vi "DataStorageCloseEventRequest_Create.vi"(7 "Header":T3, 8 "error in (no error)":errorcluster, 9 "DataStorageCloseEventRequest":T1, 10 "IRoutingSource":T2, 11 "ReplyTo":string) -> (0 "error out":errorcluster, 3 "Message":T5)   [LabVIEW 2017]
uses:
  <vilib>/addons/InsightCM/MessageBus/Base/controls/Message.ctl
  <vilib>/addons/InsightCM/MessageBus/Base/controls/MessageHeader.ctl
  <vilib>/addons/InsightCM/MessageBus/Base/controls/KeyValuePair.ctl
  <vilib>/addons/InsightCM/MessageBus/Base/controls/IRoutingSource.ctl
  <vilib>/addons/InsightCM/MessageBus/MessageLibrary/DataStorage/controls/DataStorageCloseEventRequestBody.ctl
  <vilib>/addons/InsightCM/MessageBus/Base/controls/MessageClassType.ctl
  <vilib>/addons/InsightCM/Utilities/PropertyHelpers/PropertyHelpers.lvlib
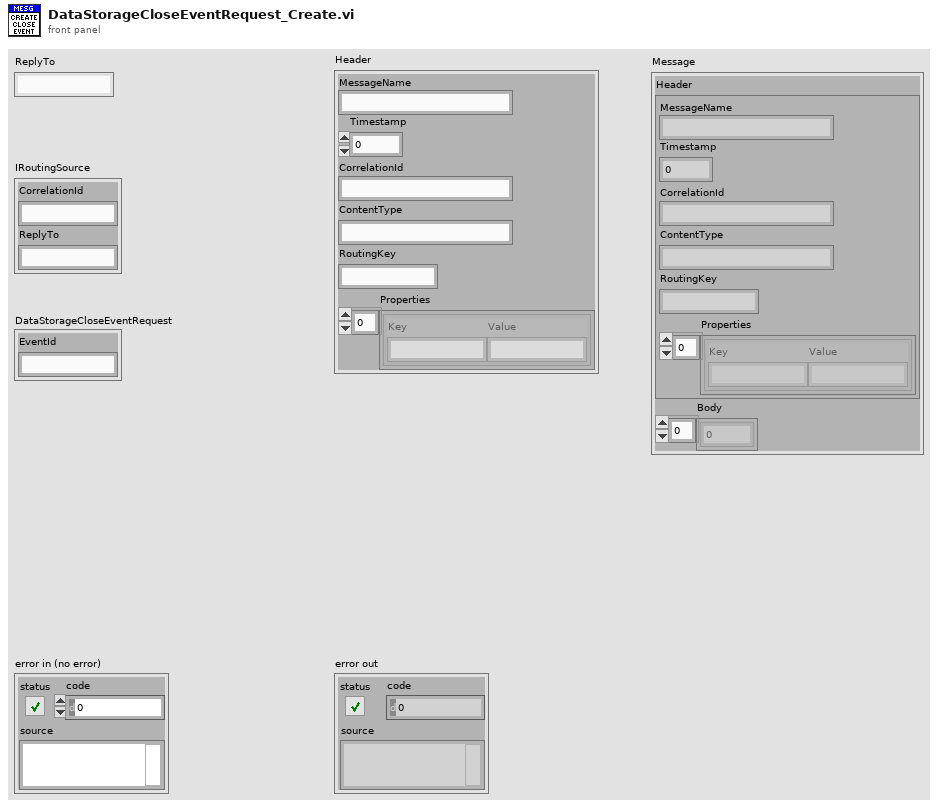
[diagram p1: front panel]
types:
  T1 = typedef "DataStorageCloseEventRequestBody.ctl" = cluster{"EventId":string}
  T2 = typedef "IRoutingSource.ctl" = cluster{"CorrelationId":string, "ReplyTo":string}
  T3 = typedef "MessageHeader.ctl" = cluster{"MessageName":string, "Timestamp":i64, "CorrelationId":string, "ContentType":string, "RoutingKey":string, "Properties":T4[]}
  T4 = typedef "KeyValuePair.ctl" = cluster{"Key":string, "Value":string}
  T5 = typedef "Message.ctl" = cluster{"Header":T3, "Body":u8[]}
  T6 = typedef "MessageClassType.ctl" = enum16{"Request", "Response", "Broadcast", "RoutedMessage"}
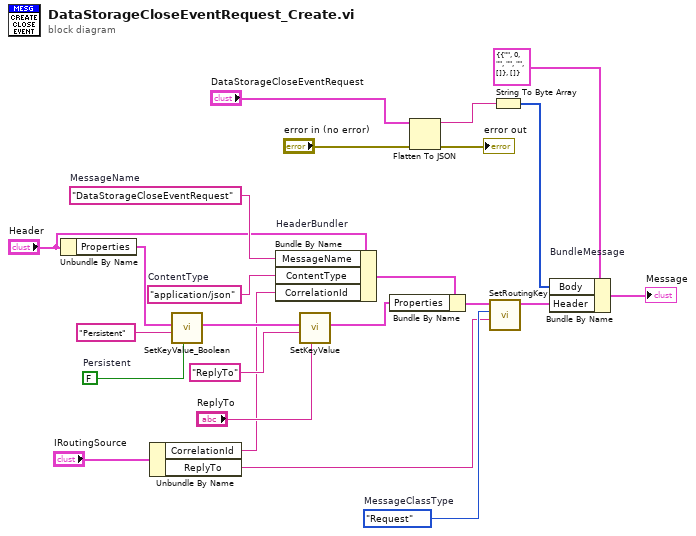
[diagram p0: block diagram]
diagram:
  w20 = MessageClassType."Request"  # MessageClassType
  w15 = FALSE  # Persistent
  w21 = "DataStorageCloseEventRequest"  # MessageName
  w18 = "application/json"  # ContentType
  n1 = Unbundle By Name("Header") -> ("Properties"=w17:T4[])
  n2 = Unbundle By Name("IRoutingSource") -> ("CorrelationId"=w4:string, "ReplyTo"=w3:string)
  n3 = call <vilib>:"SetKeyValue_Boolean.vi"("value"=w15, "key"="Persistent" ("Key"), "key value pairs"=w17) -> ("key value pairs out"=w13:T4[])  [unwired: 8 in]
  n4 = Bundle By Name "HeaderBundler"(cluster="Header", "MessageName"=w21, "ContentType"=w18, "CorrelationId"=w4) -> (w11:T3)
  n5 = call <vilib>:"SetKeyValue.vi"("value"="ReplyTo", "key"="ReplyTo" ("Key"), "key value pairs"=w13) -> ("key value pairs out"=w10:T4[])  [unwired: 8 in]
  n6 = Bundle By Name(cluster=w11, "Properties"=w10) -> (w12:T3)
  n7 = Flatten To JSON(anything="DataStorageCloseEventRequest", error in (no error)="error in (no error)") -> (JSON string=w2:string, 11:→"error out":errorcluster)  [unwired: 1 in]
  n8 = call <vilib>:"SetRoutingKey.vi"("SendTo"=w3, "MessageClassType"=w20, "Message Header in"=w12) -> ("Message Header out"=w14:T3)  [unwired: 8 in]
  n9 = String To Byte Array(string=w2) -> (unsigned byte array=w23:u8[])
  n10 = Bundle By Name "BundleMessage"(cluster=T5 {"Header"={"MessageName"="", "Timestamp"=0, "CorrelationId"="", "ContentType"="", "RoutingKey"="", "Properties"=[]}, "Body"=[]} ("Message"), "Body"=w23, "Header"=w14) -> (→"Message":T5)
